vi "Return System Session.vi"(8 "error in":errorcluster, 11 "RT Management in":refnum<class "RT Management.lvclass">) -> (0 "error out":errorcluster, 3 "RT Management out":refnum<class "RT Management.lvclass">)   [LabVIEW 2015, in "SMI.lvlib"]
uses:
  SMI.lvlib
  RT Management.lvclass
panel:
  in  "SysCfg Session":refnum<k21>
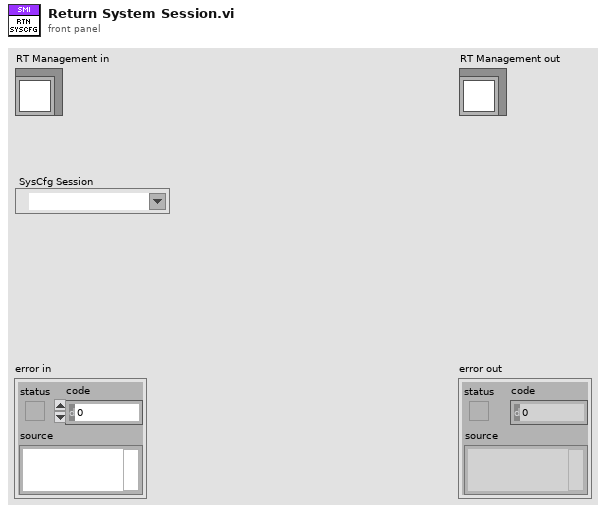
[diagram p1: front panel]
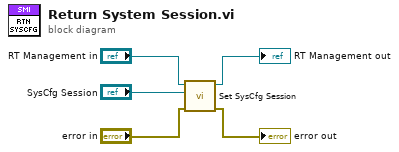
[diagram p0: block diagram]
diagram:
  n1 = call "Set SysCfg Session.vi"("error in (no error)"="error in", "SysCfg Session"="SysCfg Session", "RT Management Session in"="RT Management in") -> ("error out"=→"error out":errorcluster, "RT Management Session out"=→"RT Management out":refnum<class "RT Management.lvclass">)  [unwired: 7 in]
